vi "getTriggerSequence.vi"(8 "error in (no error)":errorcluster, 11 "Xcite in":refnum<class "Xcite.lvclass">) -> (0 "error out":errorcluster, 2 "trigger_sequence":u16[](array[numeric]), 3 "Xcite out":refnum<class "Xcite.lvclass">)   [LabVIEW 2019, in "Xcite.lvclass"]
doc: "Gets the current sequnce configuration from the X-Cite light source."
uses:
  Xcite.lvclass
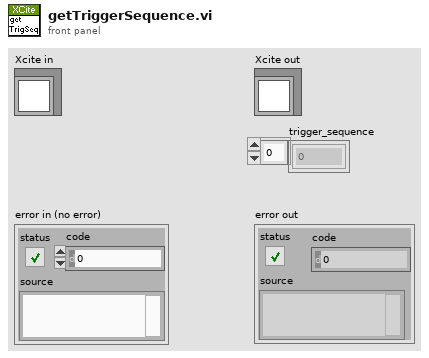
[diagram p1: front panel]
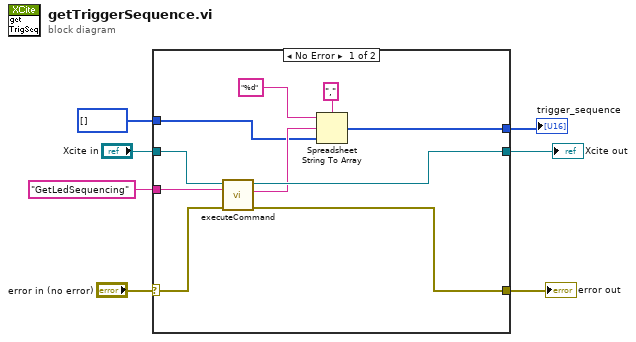
[diagram p0: block diagram]
diagram:
  n1 = case shown="No Error" "error in (no error)" {
    selector: "error in (no error)" -> [w9 w19]
    tunnel: "Xcite in" -> [w17 w20]
    tunnel: "GetLedSequencing" -> [w16 _]
    tunnel: [w15 w20] -> w5
    tunnel: [w14 w19] -> w4
    tunnel: u16[] [] -> [w10 w18]
    tunnel: [w8 w18] -> w1
    frame No Error {
      n2 = call "executeCommand.vi"("error in (no error)"=w9, "cmd"=w16, "Xcite in"=w17) -> ("error out"=w14:errorcluster, "to"=w13:string, "Xcite out"=w15:refnum<class "Xcite.lvclass">)  [unwired: 6 in]
      n3 = Spreadsheet String To Array(delimiter (Tab)=",", format string="%d", spreadsheet string=w13, array type (2D Dbl)=w10) -> (array=w8:u16[])
    }
    frame Error {
    }
  }
  "Xcite out" <- w5
  "error out" <- w4
  "trigger_sequence" <- w1
